vi "S2C_Access_Insert.vi"(8 "Error In":errorcluster, 9 "Data":variant, 10 "Columns":string[](array[string]), 11 "Table":string) -> (0 "Error Out":errorcluster)   [LabVIEW 2015]
uses:
  S2C_Access_Globals.vi
  <vilib>/addons/database/NI_Database_API.lvlib
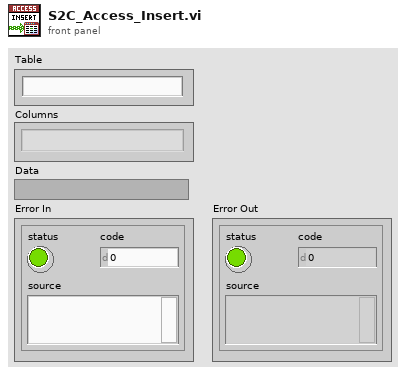
[diagram p1: front panel]
types:
  T1 = typedef "NI_Database_API.lvlib/Conn ObjectReference.ctl" = refnum<k1>
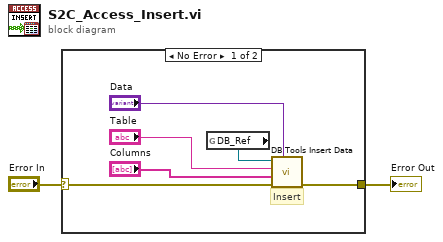
[diagram p0: block diagram]
diagram:
  n1 = case shown="No Error" "Error In" {
    selector: "Error In" -> [w8 w9]
    tunnel: [w7 w9] -> w1
    frame No Error {
      # "Insert"
      n2 = global read "S2C_Access_Globals.vi" "DB_Ref"() -> (w6:T1)
      n3 = call <vilib>:"DB Tools Insert Data.vi"("data"="Data", "error in (no error)"=w8, "columns"="Columns", "table"="Table", "connection reference"=w6) -> ("error out"=w7:errorcluster)  [unwired: 5 in, 1 out]
    }
    frame Error {
    }
  }
  "Error Out" <- w1
